vi "send PIE (with Chrip).vi"() -> ()   [LabVIEW 2017]
uses:
  <vilib>/measure/maspectr.llb/FFT Spectrum (Mag-Phase) for 1 Chan.vi
  <instrlib>/niUSRP/niUSRP Write Tx Data (CDB).vi
  <vilib>/measure/NI_MAPro.lvlib
panel:
  out "波形图 2":dbl[](graph)
  out "magnitude":cluster{"f0":dbl, "df":dbl, "magnitude":dbl[]}(graph) caption="幅度"
  in  "停止":bool
  out "波形图":dbl[](graph)
  out "error out":errorcluster
  in  "end of data?":bool
  in  "timeout":dbl=10.0
  out "coerced IQ rate":dbl=100000.0 format="%#_6p"
  out "coerced gain":dbl format="%#_6f"
  out "coerced carrier frequency":dbl=100000.0 format="%#_6p"
  in  "active antenna":string="TX1"
  in  "gain":dbl=30.0 format="%#_6f"
  in  "carrier frequency":dbl=915000000.0 format="%#_6p"
  in  "IQ rate":dbl=1000000.0 format="%#_6p"
  in  "Enabled Channels":string="0"
  in  "device names":refnum<k15>="192.168.10.10"
  out "大小":i32
  in  "输入序列":u32[](array[numeric]) format="%b"
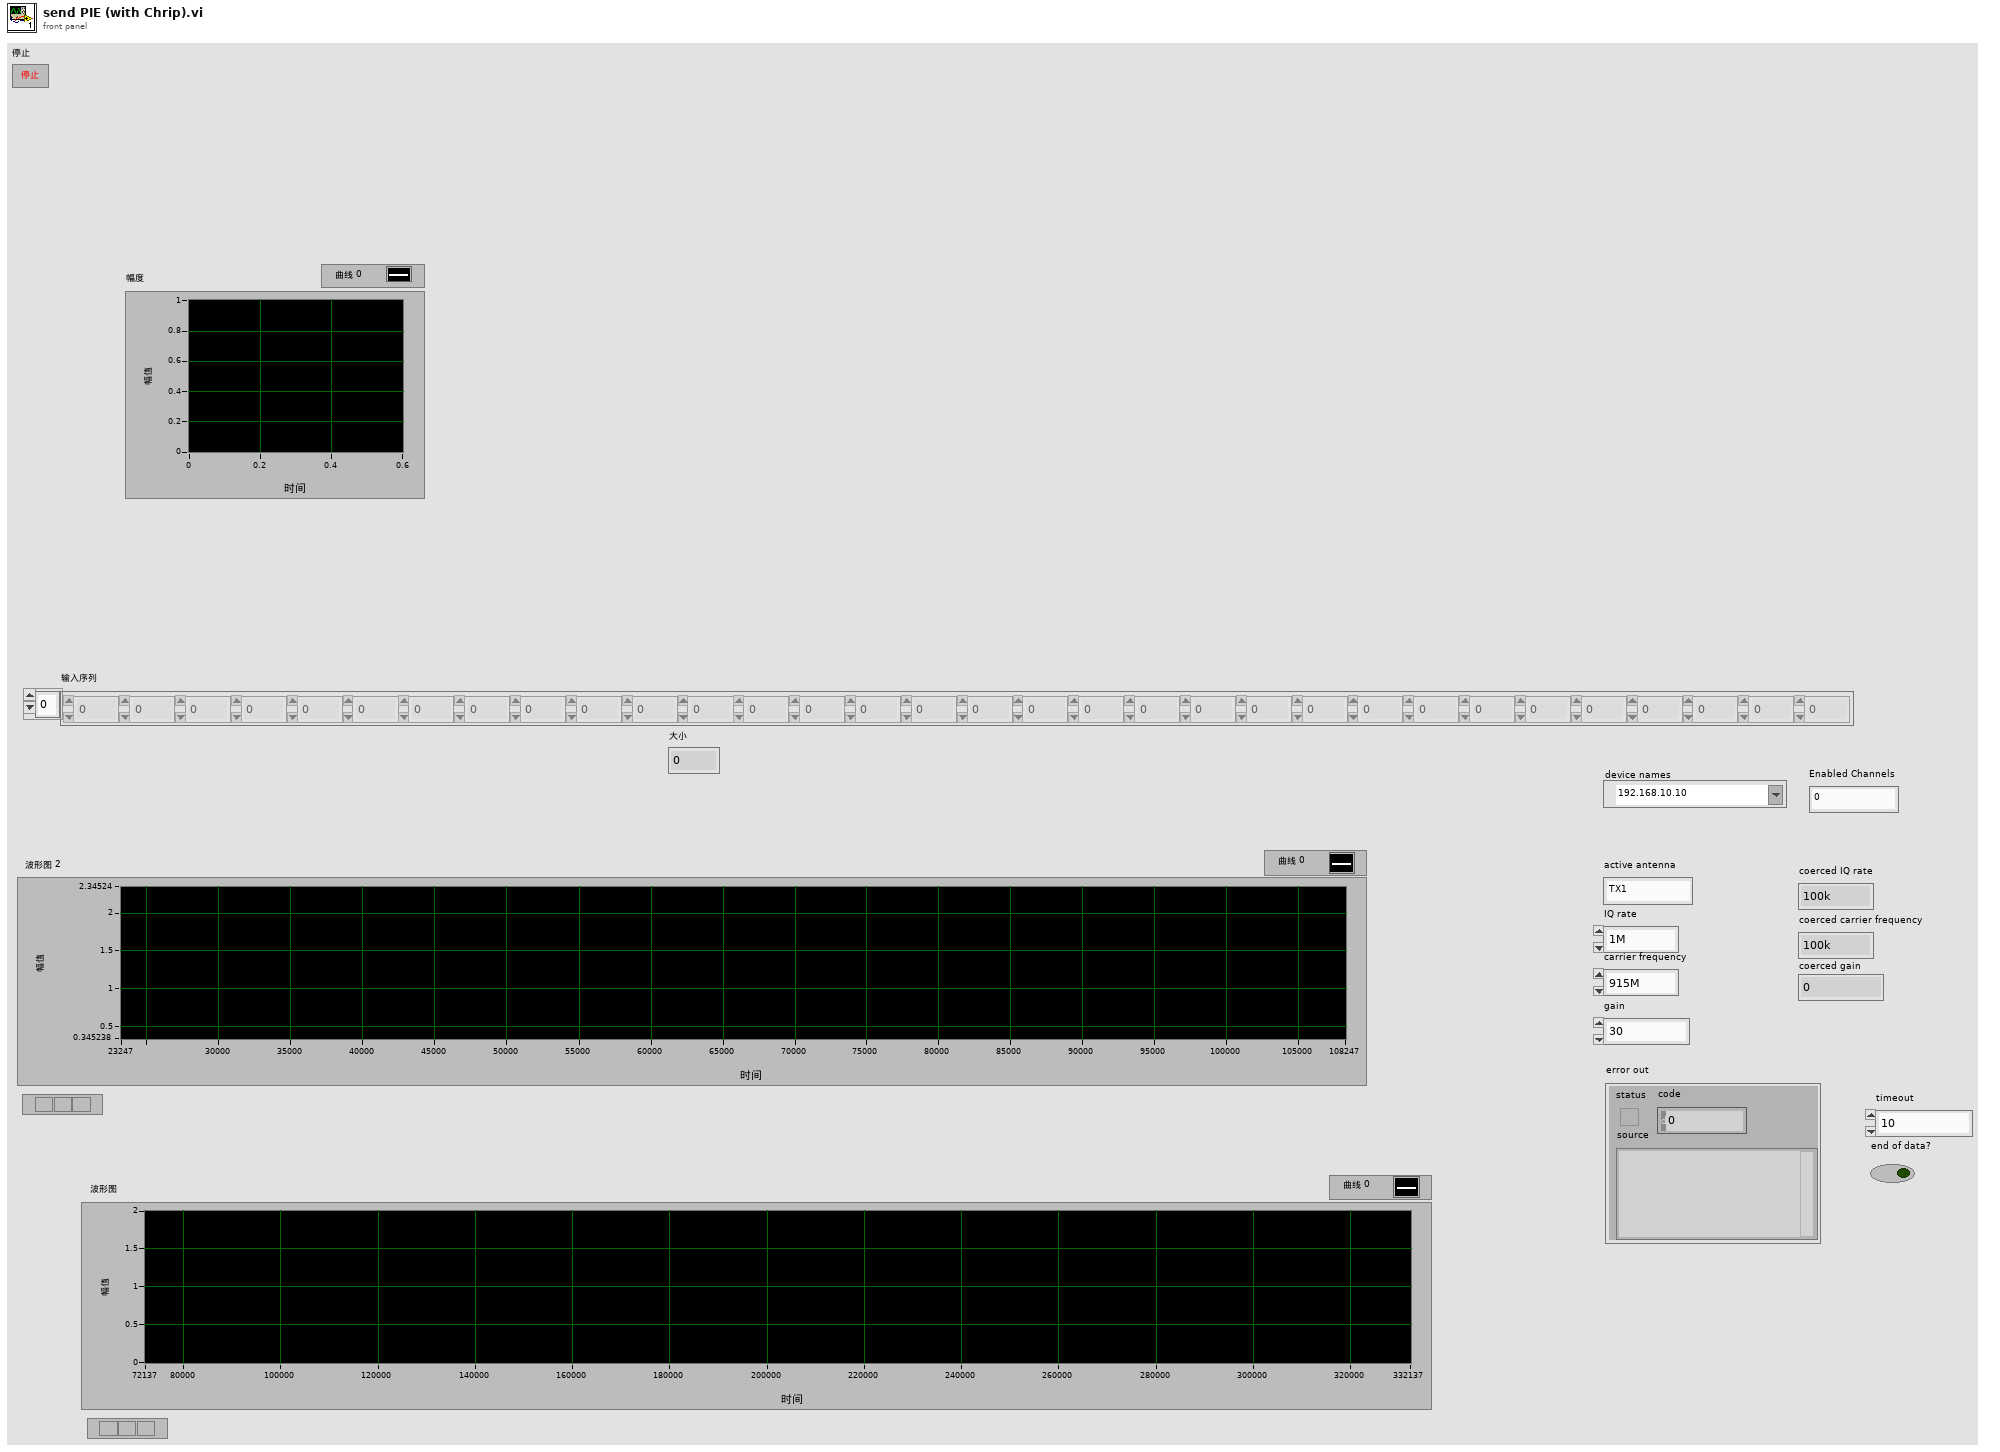
[diagram p1: front panel]
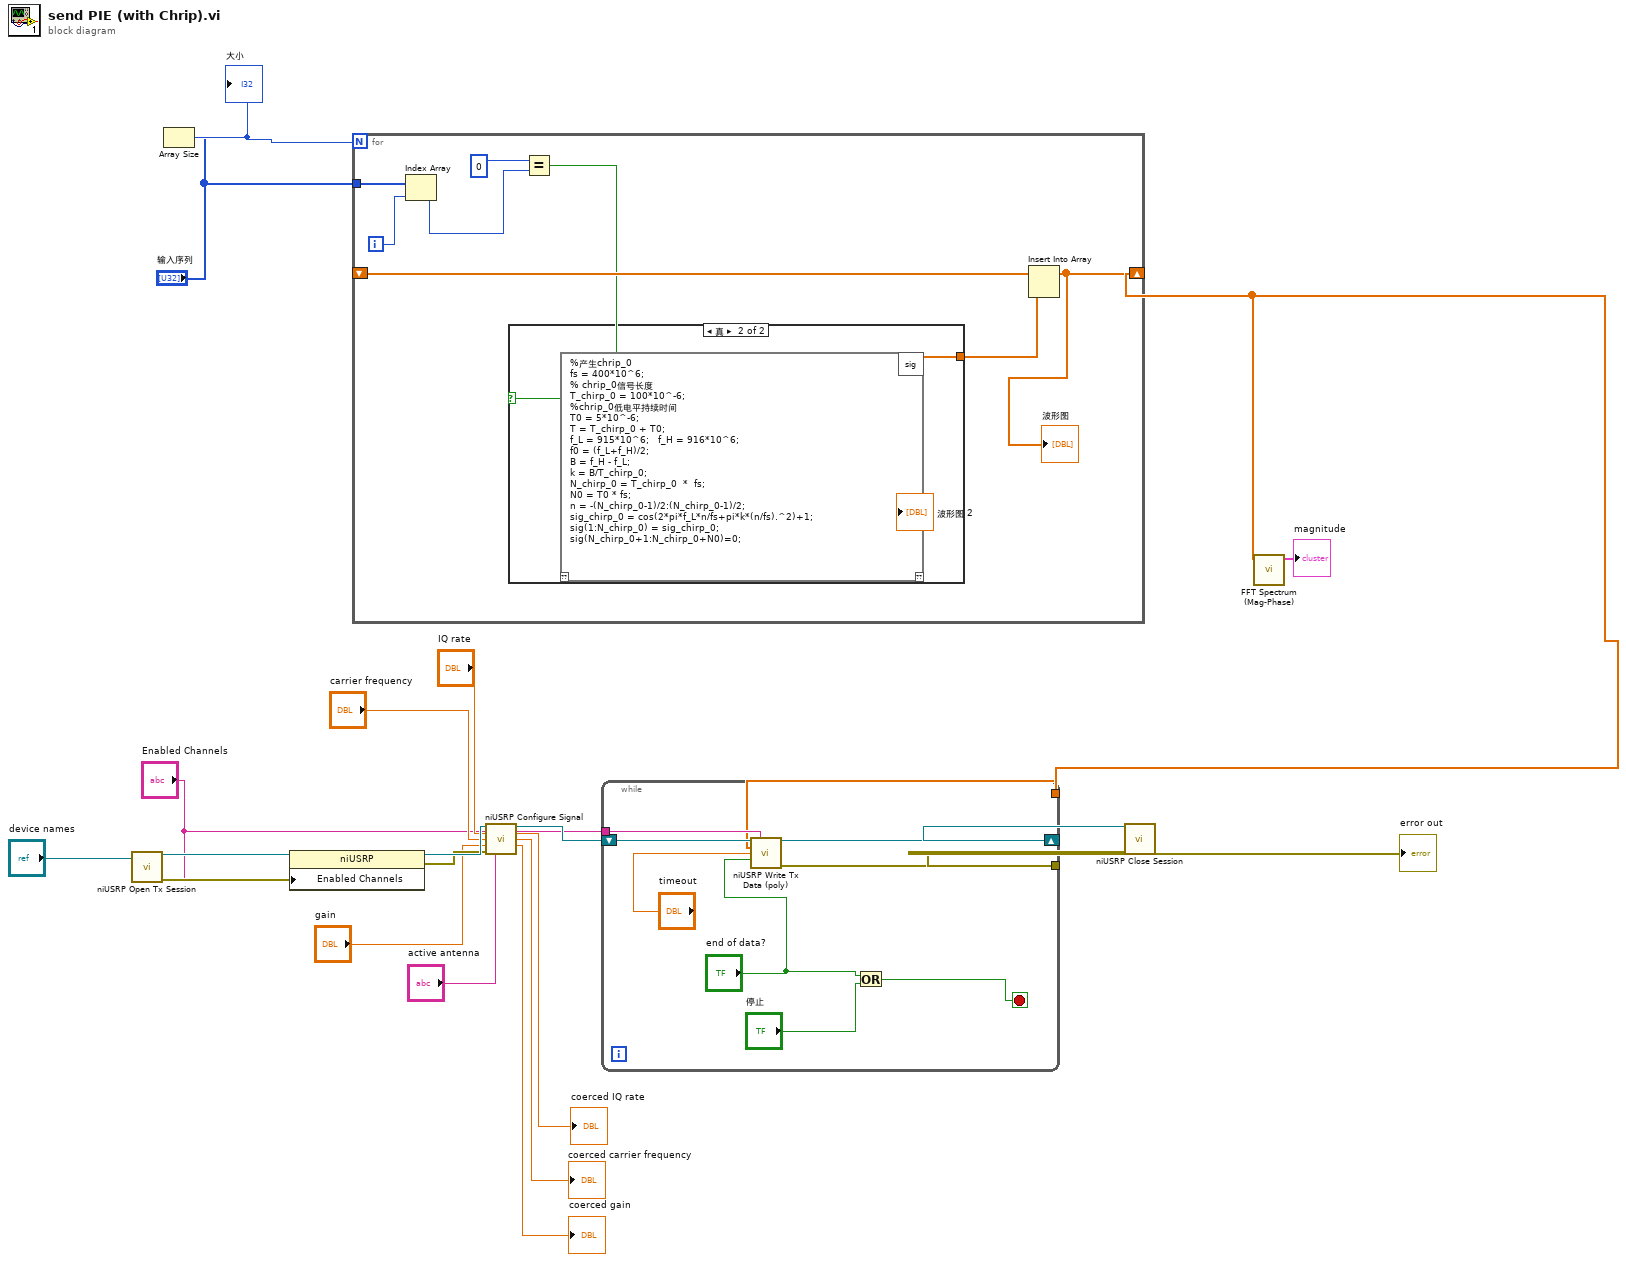
[diagram p0: block diagram]
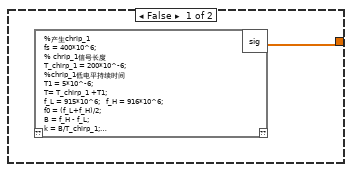
[diagram p2: hidden frame]
diagram:
  n1 = call <instrlib>:"niUSRP Open Tx Session.vi"("device names"="device names") -> ("session handle out"=w18:refnum<k15>, "error out"=w17:errorcluster)  [unwired: 13 in]
  n2 = Array Size(array="输入序列") -> (size(s)=w21:i32)
  "大小" <- w21
  n3 = property class="niUSRP"(reference=w18, error in=w17, "Enabled Channels"="Enabled Channels") -> (reference out=w16:refnum<k15>, error out=w15:errorcluster)
  n4 = for {
    N: w21 -> [_]
    tunnel: "输入序列" -> [w27]
    shift-right: [w25] -> w1
    shift-left: _ -> [w24]
    i -> [w29]
    n5 = Index Array(array=w27, index=w29) -> (element=w23:u32)
    n6 = Equal?(x=u32 0, y=w23) -> (x = y?=w22:bool)
    n7 = case shown="真" w22 {
      tunnel: [w30 w31] -> w26
      frame False {
        n8 = script code="%产生chrip_1\nfs = 400*10^6;                                               \n% chrip_1信号长度\nT_chirp_1 = 200*10^-6;      \n%chrip_1低电平持续时间\nT1 = 5*10^-6;\nT= T_chirp_1 +T1;\nf_L = 915*10^6;   f_H = 916*10^6;\nf0 = (f_L+f_H)/2;                                           \nB = f_H - f_L;\nk = B/T_chirp_1;\nN_chirp_1 = T_chirp_1 * fs;\nN1 = T1 * fs;\nn = -(N_chirp_1-1)/2:(N_chirp_1-1)/2;\nsig_chirp_0 = cos(2*pi*f0*n/fs+pi*k*(n/fs).^2)+1;\nsig(1:N_chirp_1) = sig_chirp_0;\nsig(N_chirp_1+1:N_chirp_1+N1)=0;"() -> ("sig"=w30:cdb[])  [unwired: 1 in, 1 out]
      }
      frame True {
        n9 = script code="%产生chrip_0\nfs = 400*10^6; \n% chrip_0信号长度\nT_chirp_0 = 100*10^-6;      \n%chrip_0低电平持续时间\nT0 = 5*10^-6;\nT = T_chirp_0 + T0;\nf_L = 915*10^6;   f_H = 916*10^6;\nf0 = (f_L+f_H)/2;                                           \nB = f_H - f_L;\nk = B/T_chirp_0;\nN_chirp_0 = T_chirp_0  *  fs;\nN0 = T0 * fs;\nn = -(N_chirp_0-1)/2:(N_chirp_0-1)/2;\nsig_chirp_0 = cos(2*pi*f_L*n/fs+pi*k*(n/fs).^2)+1;\nsig(1:N_chirp_0) = sig_chirp_0;\nsig(N_chirp_0+1:N_chirp_0+N0)=0;"() -> ("sig"=w31:cdb[])  [unwired: 1 in, 1 out]
        "波形图 2" <- w31
      }
    }
    n10 = Insert Into Array(array=w24, new element=w26) -> (w25:cdb[])  [unwired: 1 in]
    "波形图" <- w25
  }
  n11 = call <instrlib>:"niUSRP Configure Signal.vi"("session handle"=w16, "channel list"="Enabled Channels", "IQ rate"="IQ rate", "carrier frequency"="carrier frequency", "gain"="gain", "error in (no error)"=w15, "active antenna"="active antenna") -> ("session handle out"=w7:refnum<k15>, "coerced IQ rate"=→"coerced IQ rate":dbl, "coerced carrier frequency"=→"coerced carrier frequency":dbl, "coerced gain"=→"coerced gain":dbl)  [unwired: 4 in, 1 out]
  n12 = while {
    tunnel: "Enabled Channels" -> [w39]
    tunnel: [w36] -> w3
    tunnel: w1 -> [w35]
    shift-right: [w37] -> w4
    shift-left: w7 -> [w40]
    stop <- w32 stop-if-true
    n13 = call-poly <instrlib>:"niUSRP Write Tx Data (poly).vi"("session handle"=w40, "channel list"=w39, "data"=w35, "timeout"="timeout", "end of data?"="end of data?") -> ("session handle out"=w37:refnum<k15>, "error out"=w36:errorcluster)  [unwired: 9 in]
    n14 = Or(x="end of data?", y="停止") -> (x .or. y?=w32:bool)
  }
  n15 = call <instrlib>:"niUSRP Close Session.vi"("session handle"=w4, "error in (no error)"=w3) -> ("error out"=→"error out":errorcluster)  [unwired: 13 in]
  n16 = call-poly <vilib>:"FFT Spectrum (Mag-Phase).vi"("time signal"=w1) -> ("magnitude"=→"magnitude":cluster{"f0":dbl, "df":dbl, "magnitude":dbl[]})  [unwired: 6 in, 4 out]
